vi "main(with error).vi"() -> ()   [LabVIEW 2013]
uses:
  src/_gStop.vi
  src/GlobalStop(dev).lvlib
panel:
  in  "gen error":bool
  out "error out":errorcluster
  out "loop4":i32
  in  "stop 2":bool
  out "loop3":i32
  out "loop2":i32
  out "loop1":i32
  in  "stop":bool
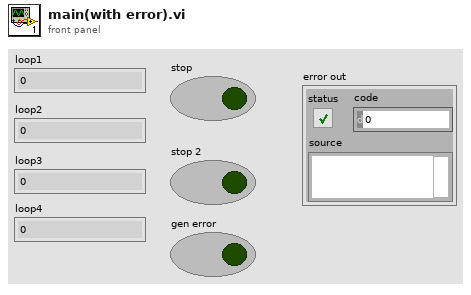
[diagram p1: front panel]
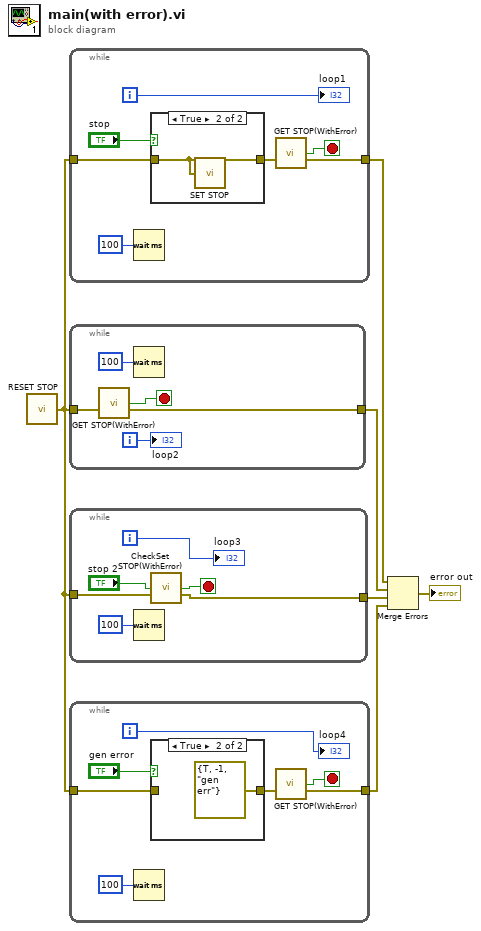
[diagram p0: block diagram]
diagram:
  n1 = call "RESET STOP.vi"() -> ("error out"=w3:errorcluster)  [unwired: 5 in]
  n2 = while {
    tunnel: w3 -> [w13]
    tunnel: [w7] -> w6
    i -> [w11]
    stop <- w8 stop-if-true
    n3 = Wait (ms)(milliseconds to wait=100) -> ()  [unwired: 1 out]
    n4 = case shown="True" "stop" {
      tunnel: w13 -> [w14 w15]
      tunnel: [w14 w15] -> w9
      frame False {
      }
      frame True {
        n5 = call "SET STOP.vi"("error in (no error)"=w15) -> ()  [unwired: 4 in, 1 out]
      }
    }
    n6 = call "GET STOP(WithError).vi"("error in (no error)"=w9) -> ("Stop"=w8:bool, "error out"=w7:errorcluster)  [unwired: 13 in]
    "loop1" <- w11
  }
  n7 = while {
    tunnel: w3 -> [w18]
    tunnel: [w16] -> w5
    i -> [w20]
    stop <- w17 stop-if-true
    n8 = call "GET STOP(WithError).vi"("error in (no error)"=w18) -> ("Stop"=w17:bool, "error out"=w16:errorcluster)  [unwired: 13 in]
    n9 = Wait (ms)(milliseconds to wait=100) -> ()  [unwired: 1 out]
    "loop2" <- w20
  }
  n10 = while {
    tunnel: w3 -> [w23]
    tunnel: [w22] -> w4
    i -> [w26]
    stop <- w21 stop-if-true
    n11 = Wait (ms)(milliseconds to wait=100) -> ()  [unwired: 1 out]
    n12 = call "CheckSet STOP(WithError).vi"("stop value"="stop 2", "error in (no error)"=w23) -> ("Boolean"=w21:bool, "error out"=w22:errorcluster)  [unwired: 12 in]
    "loop3" <- w26
  }
  n13 = while {
    tunnel: w3 -> [w30]
    tunnel: [w28] -> w2
    i -> [w33]
    stop <- w27 stop-if-true
    n14 = Wait (ms)(milliseconds to wait=100) -> ()  [unwired: 1 out]
    n15 = case shown="True" "gen error" {
      tunnel: w30 -> [w34 _]
      tunnel: [w34 errorcluster {"status"=TRUE, "code"=-1, "source"="gen err"} ("error out")] -> w29
      frame False {
      }
      frame True {
      }
    }
    n16 = call "GET STOP(WithError).vi"("error in (no error)"=w29) -> ("Stop"=w27:bool, "error out"=w28:errorcluster)  [unwired: 13 in]
    "loop4" <- w33
  }
  n17 = Merge Errors(w6, w5, w4, w2) -> (→"error out":errorcluster)
